vi "AO Parameter.vi"(8 "error in (no error)":errorcluster, 11 "Node Ptr":T1 format="%.0x") -> (0 "error out":errorcluster)   [LabVIEW 2023, in "Waveform Analog Output System Explorer.lvlib"]
uses:
  Waveform Analog Output System Explorer.lvlib
  <vilib>/NI VeriStand/Custom Device API/Custom Device Item Ref.ctl
  NationalInstruments.VeriStand.SystemDefinitionAPI
  <vilib>/NI VeriStand/Custom Device API/Custom Device API.lvlib
panel:
  out "Channel Settings":i32(listbox)
  in  "Default Value":dbl
  in  "Header":cluster{"Section Name":string}={"Section Name"="Custom Device Channel Specification"}
  in  "Description":string
  in  "Name":string
  # "This is custom"
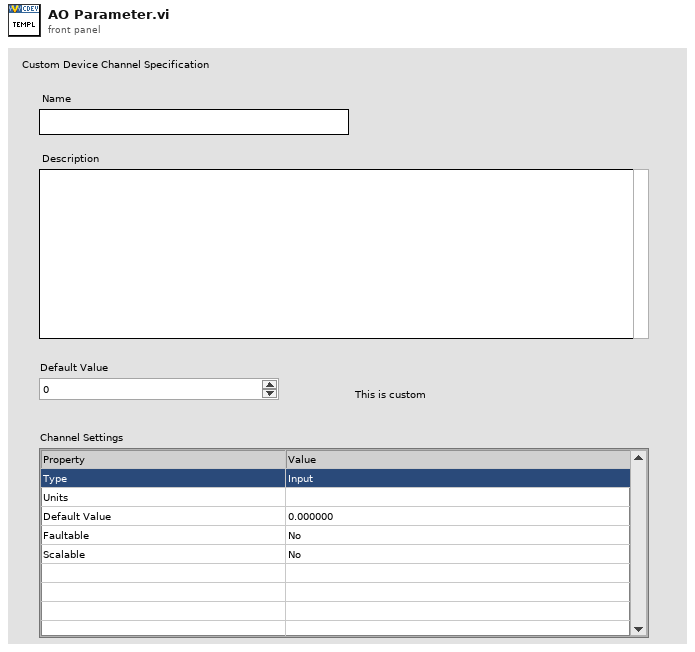
[diagram p1: front panel]
types:
  T1 = typedef "Custom Device API.lvlib/Custom Device Item Ref.ctl" = u64
  T2 = typedef "Custom Device API.lvlib/Custom Device Item Info.ctl" = cluster{"Name":string, "Is Channel":bool, "GUID":string, "Is Waveform":bool}
  T3 = typedef "Custom Device API.lvlib/Custom Device Pointer.ctl" = refnum<k24>
  T4 = typedef "Custom Device API.lvlib/Custom Device Commands.ctl" = enum16{"Default", "Item renamed", "Shutdown", "Dynamic button pressed"}
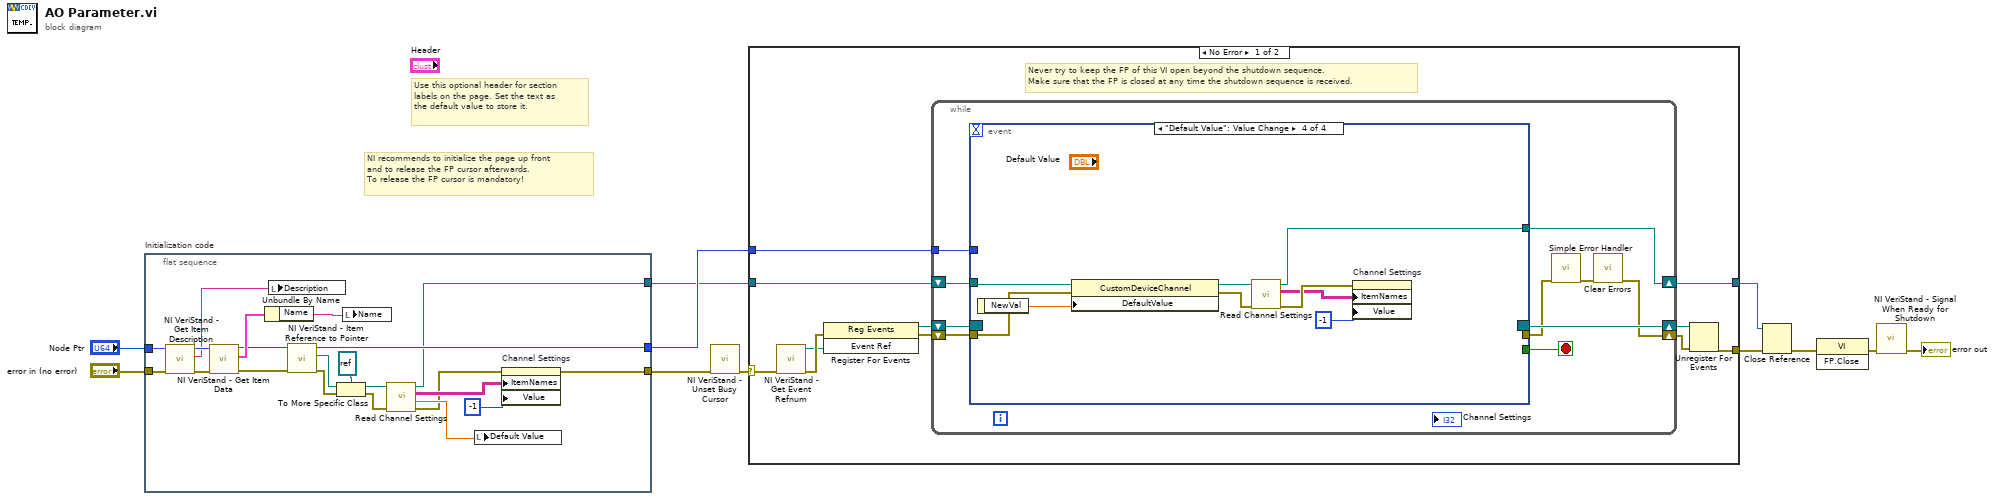
[diagram p0: block diagram]
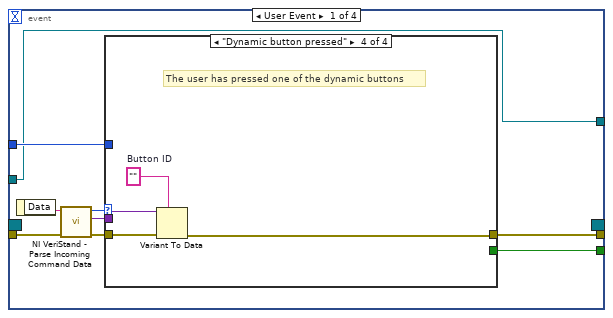
[diagram p2: hidden frame]
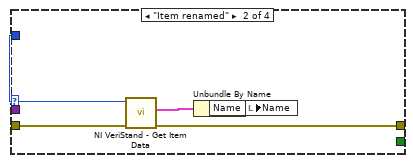
[diagram p4: hidden frame]
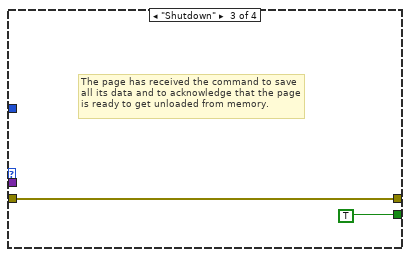
[diagram p5: hidden frame]
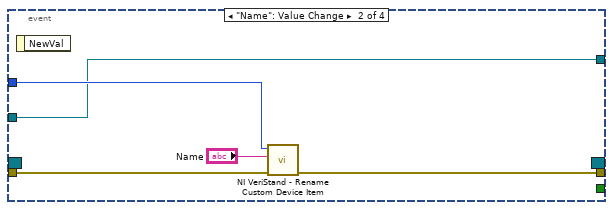
[diagram p6: hidden frame]
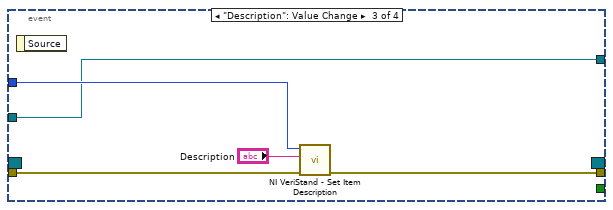
[diagram p7: hidden frame]
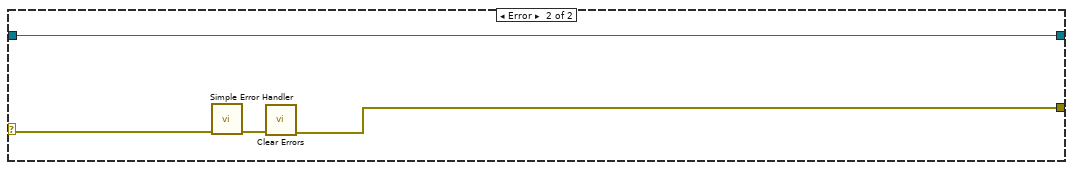
[diagram p8: hidden frame]
diagram:
  # "Use this optional header for section labels on the page. Set the text as the default value to store it."
  # "NI recommends to initialize the page up front\nand to release the FP cursor afterwards.\nTo release the FP cursor is mandatory!"
  n1 = flat-sequence "Initialization code" {
    tunnel: "error in (no error)" -> [w31]
    tunnel: "Node Ptr" -> [w30]
    tunnel: [w23] -> w6
    tunnel: [w15] -> w5
    tunnel: [w19] -> w4
    frame #0 {
      n2 = call <vilib>:"NI VeriStand - Get Item Description.vi"("error in (no error)"=w31, "Item Ref in"=w30) -> ("error out"=w29:errorcluster, "Description"=w26:string, "Item Ref out"=w32:T1)  [unwired: 7 out]
      n3 = call <vilib>:"NI VeriStand - Get Item Data.vi"("error in (no error)"=w29, "Item Ref in"=w32) -> ("error out"=w24:errorcluster, "Item Info"=w28:T2, "Item Ref out"=w25:T1)  [unwired: 7 out]
      n4 = Unbundle By Name(w28) -> ("Name"=w27:string)
      n5 = local write "Description"(w26) -> ()
      n6 = call <vilib>:"NI VeriStand - Item Reference to Pointer.vi"("error in (no error)"=w24, "Item Ref in"=w25) -> ("error out"=w13:errorcluster, "Node Pointer"=w12:T3, "Item Ref out"=w23:T1)  [unwired: 6 in, 1 out]
      n7 = To More Specific Class(target class=refnum<k24> refnum, reference=w12, error in=w13) -> (specific class reference=w21:refnum<k24>, error out=w20:errorcluster)
      n8 = local write "Name"(w27) -> ()
      n9 = call "Read Channel Settings.vi"("error in (no error)"=w20, ".NET Refnum in"=w21) -> ("error out"=w16:errorcluster, "DefaultValue"=w18:dbl, "Array"=w17:string[][], ".NET Refnum out"=w19:refnum<k24>)  [unwired: 6 in]
      n10 = local write "Default Value"(w18) -> ()
      n11 = property on="Channel Settings" class="MCListbox (strict)"(error in=w16, "ItemNames"=w17, "Value"=-1 ("Channel Settings")) -> (error out=w15:errorcluster)  [unwired: 1 in, 1 out]
    }
  }
  n12 = call <vilib>:"NI VeriStand - Unset Busy Cursor.vi"("error in (no error)"=w5) -> ("error out"=w8:errorcluster)  [unwired: 10 out]
  n13 = case shown="No Error" w8 {
    selector: w8 -> [w35 w97]
    tunnel: [w40 w95] -> w3
    tunnel: w6 -> [w36 _]
    tunnel: w4 -> [w34 w94]
    tunnel: [w33 w94] -> w2
    frame No Error {
      # "Never try to keep the FP of this VI open beyond the shutdown sequence.\nMake sure that the FP is closed at any time the shutdown sequence is received."
      n14 = call <vilib>:"NI VeriStand - Get Event Refnum.vi"("error in (no error)"=w35) -> ("error out"=w43:errorcluster, "Event Ref"=w39:refnum<user-event>)  [unwired: 9 out]
      n15 = register-events(error in=w43, w39) -> (reference out=w37:refnum<event-registration>, error out=w38:errorcluster)  [unwired: 1 in]
      n16 = while {
        tunnel: w36 -> [w49]
        shift-right: [w46] -> w41
        shift-left: w38 -> [w52]
        shift-right: [w53] -> w42
        shift-left: w37 -> [w51]
        shift-right: [w44] -> w33
        shift-left: w34 -> [w45]
        stop <- w50 stop-if-true
        n17 = event shown="[3] \"Default Value\": Value Change" {
          selector: w51 -> [_ _ _ _]
          dyn-events: [_ _ _ _] -> w53
          timeout: _ -> [_ _ _ _]
          tunnel: w52 -> [w62 w79 w83 w92]
          tunnel: [w58 _ _ _] -> w50
          tunnel: [w57 w78 w82 _] -> w48
          tunnel: w49 -> [w56 w77 w84 _]
          tunnel: w45 -> [w54 w75 w80 w93]
          tunnel: [w54 w75 w80 w85] -> w44
          event User Event {
            n18 = event-data() -> ("Data"=w61:string)  [unwired: 1 out]
            n19 = call <vilib>:"NI VeriStand - Parse Incoming Command Data.vi"("error in (no error)"=w62, "Incoming data"=w61) -> ("error out"=w60:errorcluster, "Outgoing data"=w55:variant, "Action"=w59:T4)  [unwired: 7 out]
            n20 = case shown="\"Dynamic button pressed\"" w59 {
              tunnel: w60 -> [w63 w68 w69 w74]
              tunnel: [_ _ TRUE _] -> w58
              tunnel: [w63 w65 w69 w71] -> w57
              tunnel: w56 -> [_ w67 _ _]
              tunnel: w55 -> [_ _ _ w73]
              frame "Default", Default {
              }
              frame "Item renamed" {
                n21 = call <vilib>:"NI VeriStand - Get Item Data.vi"("error in (no error)"=w68, "Item Ref in"=w67) -> ("error out"=w65:errorcluster, "Item Info"=w66:T2)  [unwired: 8 out]
                n22 = Unbundle By Name(w66) -> ("Name"=w64:string)
                n23 = local write "Name"(w64) -> ()
              }
              frame "Shutdown" {
                # "The page has received the command to save all its data and to acknowledge that the page is ready to get unloaded from memory."
              }
              frame "Dynamic button pressed" {
                w72 = ""  # Button ID
                # "The user has pressed one of the dynamic buttons"
                n24 = Variant To Data(error in=w74, type=w72, Variant=w73) -> (error out=w71:errorcluster)  [unwired: 1 out]
              }
            }
          }
          event "Name": Value Change {
            n25 = event-data() -> ()  [unwired: 2 out]
            n26 = call <vilib>:"NI VeriStand - Rename Custom Device Item.vi"("error in (no error)"=w79, "New Name"="Name", "Item Ref in"=w77) -> ("error out"=w78:errorcluster)  [unwired: 1 in, 7 out]
          }
          event "Description": Value Change {
            n27 = event-data() -> ()  [unwired: 2 out]
            n28 = call <vilib>:"NI VeriStand - Set Item Description.vi"("error in (no error)"=w83, "Description"="Description", "Item Ref in"=w84) -> ("error out"=w82:errorcluster)  [unwired: 8 out]
          }
          event "Default Value": Value Change {
            n29 = event-data() -> ("NewVal"=w91:dbl)  [unwired: 1 out]
            n30 = property class="CustomDeviceChannel"(reference=w93, error in=w92, "DefaultValue"=w91) -> (reference out=w90:refnum<k24>, error out=w89:errorcluster)
            n31 = call "Read Channel Settings.vi"("error in (no error)"=w89, ".NET Refnum in"=w90) -> ("error out"=w88:errorcluster, "Array"=w87:string[][], ".NET Refnum out"=w85:refnum<k24>)  [unwired: 6 in, 1 out]
            n32 = property on="Channel Settings" class="MCListbox (strict)"(error in=w88, "ItemNames"=w87, "Value"=-1 ("Channel Settings")) -> ()  [unwired: 1 in, 2 out]
          }
        }
        n33 = call <vilib>:"Simple Error Handler.vi"("error in (no error)"=w48) -> ("error out"=w47:errorcluster)  [unwired: 1 in, 7 out]
        n34 = call <vilib>:"Clear Errors.vi"("error in (no error)"=w47) -> ("error out"=w46:errorcluster)  [unwired: 1 in, 5 out]
      }
      n35 = Unregister For Events(event registration refnum=w42, error in=w41) -> (error out=w40:errorcluster)
    }
    frame Error {
      n36 = call <vilib>:"Simple Error Handler.vi"("error in (no error)"=w97) -> ("error out"=w96:errorcluster)  [unwired: 1 in, 7 out]
      n37 = call <vilib>:"Clear Errors.vi"("error in (no error)"=w96) -> ("error out"=w95:errorcluster)  [unwired: 1 in, 5 out]
    }
  }
  n38 = Close Reference(reference=w2, error in (no error)=w3) -> (error out=w1:errorcluster)
  n39 = invoke class="VI" method="FP.Close"(error in=w1) -> (error out=w11:errorcluster)  [unwired: 2 in, 2 out]
  n40 = call <vilib>:"NI VeriStand - Signal When Ready for Shutdown.vi"("error in (no error)"=w11) -> ("error out"=→"error out":errorcluster)  [unwired: 10 out]
